vi "mightex.vi"() -> ()   [LabVIEW 2016]
uses:
  lib/SSClassic_USBCamera_SDK.dll
panel:
  in  "sharp":i32 min=0 max=3
  in  "bright":i32=50 min=0 max=100
  in  "contrast":i32=50 min=0 max=100
  in  "gamma":i32=10 min=1 max=20
  in  "Gain?":bool
  in  "Blue Gain":i32(slide)=17 scale=1.0..64.0
  in  "Green Gain":i32(slide)=16 scale=1.0..64.0
  in  "Red Gain":i32(slide)=20 scale=1.0..64.0
  out "new picture":picture
  out "Spectrum":u8[](graph)
  out "?":u8[](array[numeric])
  in  "STOP":bool
  in  "Exposure Time:":dbl(slide) scale=1.0..100.0
  out "ET Labelµ":dbl format="%#_3g"
  out "OK to run":bool
  out "SerialNo:":string
  out "ModuleNo:":string
  # "(ms )"
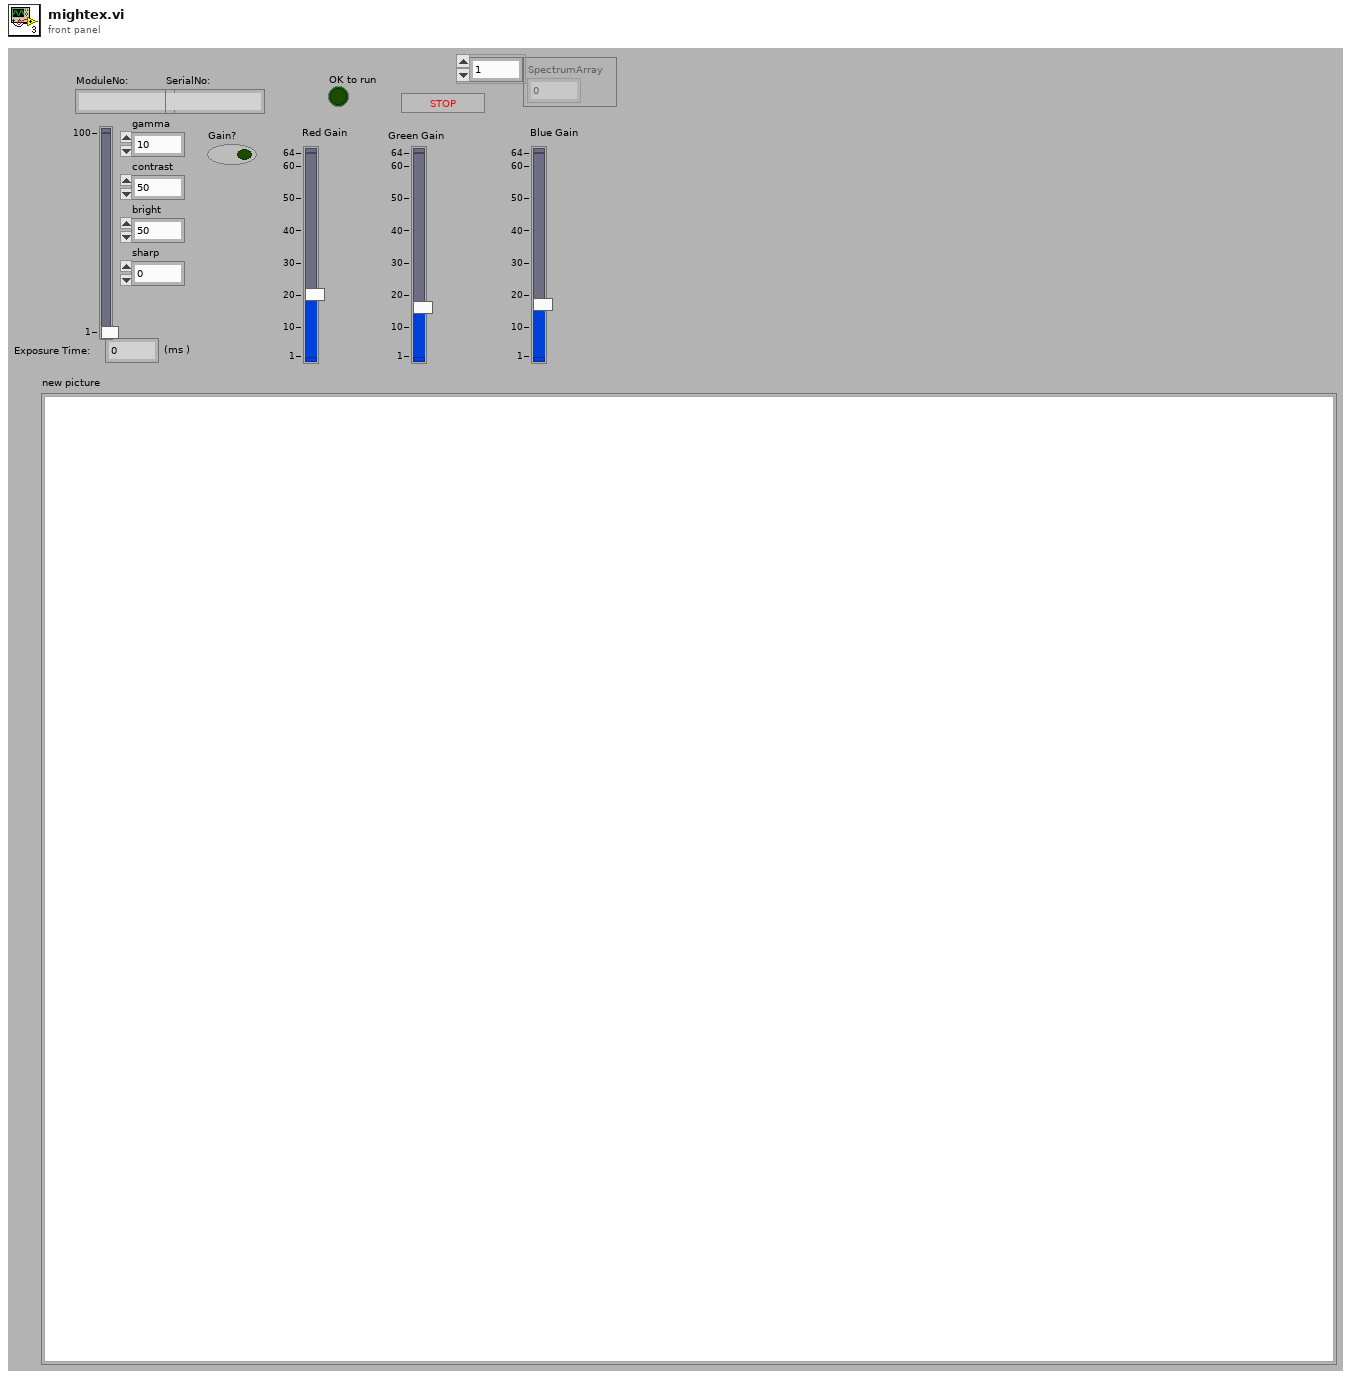
[diagram p1: front panel]
types:
  T1 = typedef "imagedata.ctl" = cluster{"image type":i32, "image depth":i32, "image":u8[], "mask":u8[], "colors":u32[], "Rectangle":cluster{"left":i16, "top":i16, "right":i16, "bottom":i16}}
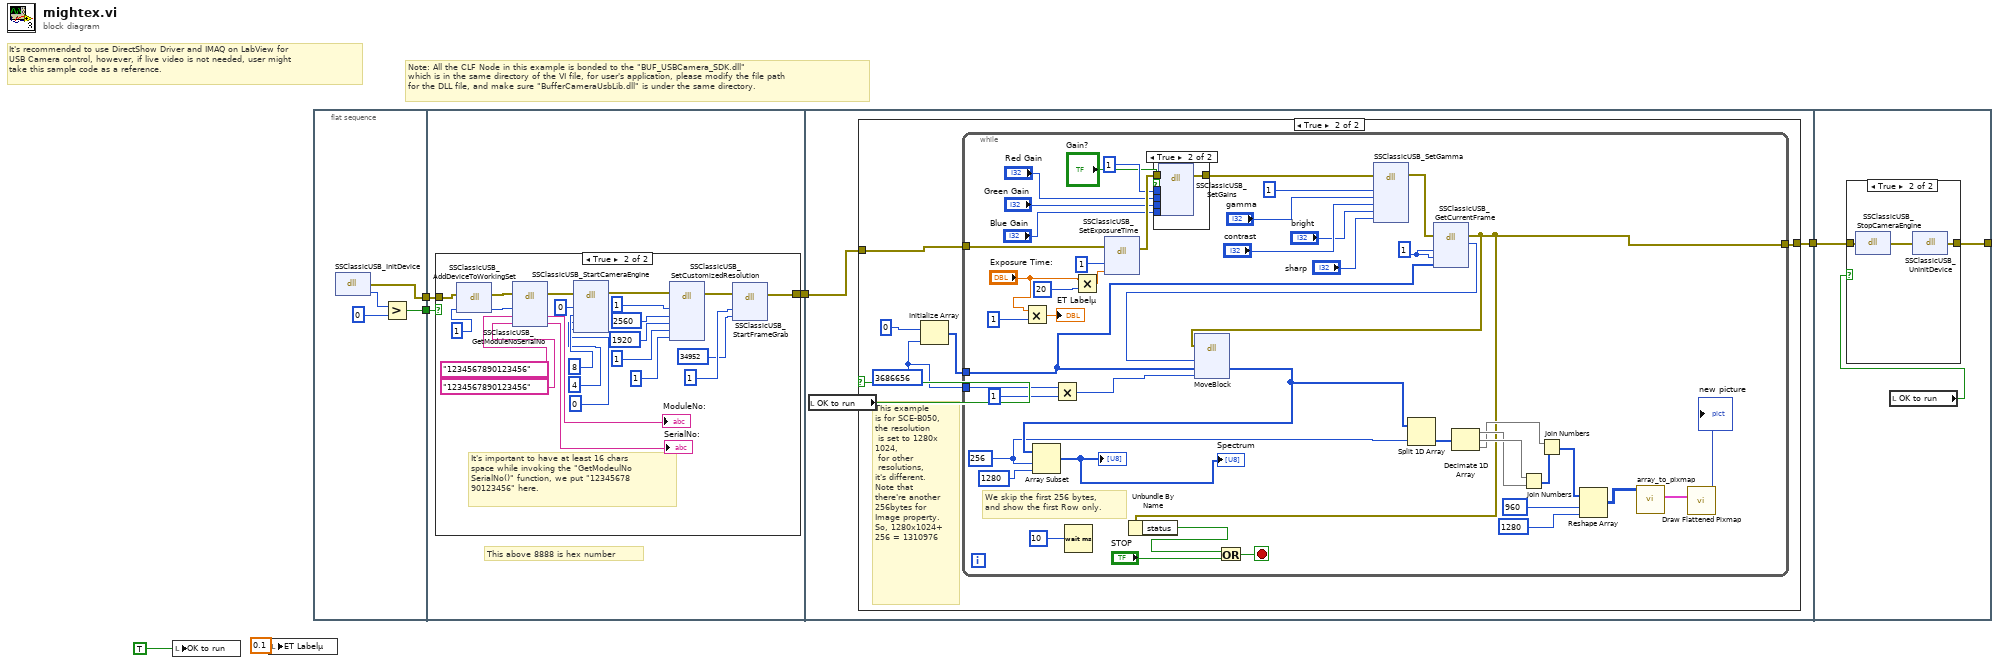
[diagram p0: block diagram]
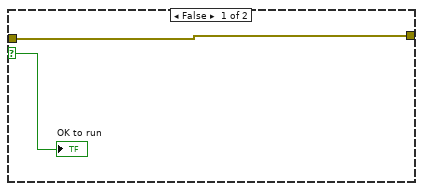
[diagram p2: hidden frame]
diagram:
  # "It's recommended to use DirectShow Driver and IMAQ on LabView for\nUSB Camera control, however, if live video is not needed, user might\ntake this sample code as a reference."
  # "Note: All the CLF Node in this example is bonded to the \"BUF_USBCamera_SDK.dll\" \nwhich is in the same directory of the VI file, for user's application, please modify the file path\nfor the DLL file, and make sure \"BufferCameraUsbLib.dll\" is under the same directory."
  n1 = local write "OK to run"(TRUE) -> ()
  n2 = local write "ET Labelµ"(0.1) -> ()
  n3 = flat-sequence {
    tunnel: [w8] -> w6
    tunnel: [w7] -> w5
    tunnel: w6 -> [w13]
    tunnel: w5 -> [w12]
    tunnel: [w11] -> w3
    tunnel: w3 -> [w40]
    tunnel: [w39] -> w2
    tunnel: w2 -> [w103]
    tunnel: [w102] -> _
    frame #0 {
      n4 = dll-call lib="D:/All users/PoSheng/src/lib/SSClassic_USBCamera_SDK.dll" fn="SSClassicUSB_InitDevice" ("CCD_USBCamera_SDK.dll:CCDUSB_InitDevice")() -> (error out=w7:errorcluster, "ReturnValue"=w10:u32)  [unwired: 3 in, 1 out]
      n5 = Greater?(x=w10, y=0) -> (0:w8:bool)
    }
    frame #1 {
      # "This above 8888 is hex number"
      n6 = case shown="True" w13 {
        selector: w13 -> [w15 _]
        tunnel: w12 -> [w14 w38]
        tunnel: [w14 w31] -> w11
        frame False {
          "OK to run" <- w15
        }
        frame True {
          # "It's important to have at least 16 chars\nspace while invoking the \"GetModeulNo\nSerialNo()\" function, we put \"12345678\n90123456\" here."
          n7 = dll-call lib="D:/All users/PoSheng/src/lib/SSClassic_USBCamera_SDK.dll" fn="SSClassicUSB_AddDeviceToWorkingSet" ("CCD_USBCamera_SDK.dll:CCDUSB_AddDeviceToWorkingSet")(error in=w38, "Arg1"=1) -> (error out=w37:errorcluster, "Arg1"=w35:i32)  [unwired: 3 in, 1 out]
          n8 = dll-call lib="D:/All users/PoSheng/src/lib/SSClassic_USBCamera_SDK.dll" fn="SSClassicUSB_GetModuleNoSerialNo" ("CCD_USBCamera_SDK.dll:CCDUSB_GetModuleNoSerialNo")(error in=w37, "Arg1"=w35, "Arg2"="1234567890123456", "Arg3"="1234567890123456") -> (error out=w33:errorcluster, "Arg2"=→"ModuleNo:":string, "Arg3"=→"SerialNo:":string)  [unwired: 4 in, 1 out]
          n9 = dll-call lib="D:/All users/PoSheng/src/lib/SSClassic_USBCamera_SDK.dll" fn="SSClassicUSB_StartCameraEngine" ("CCD_USBCamera_SDK.dll:CCDUSB_StartCameraEngine")(error in=w33, "Arg1"=0, "Arg2"=8, "Arg3"=4, "Arg4"=0) -> (error out=w26:errorcluster)  [unwired: 7 in, 1 out]
          n10 = dll-call lib="D:/All users/PoSheng/src/lib/SSClassic_USBCamera_SDK.dll" fn="SSClassicUSB_SetCustomizedResolution" ("BUF_USBCamera_SDK.dll:BUFUSB_SetCustomizedResolution")(error in=w26, "Arg1"=1, "Arg2"=2560, "Arg3"=1920, "Arg4"=1, "Arg5"=u32 1) -> (error out=w25:errorcluster)  [unwired: 8 in, 1 out]
          n11 = dll-call lib="D:/All users/PoSheng/src/lib/SSClassic_USBCamera_SDK.dll" fn="SSClassicUSB_StartFrameGrab" ("CCD_USBCamera_SDK.dll:CCDUSB_StartFrameGrab")(error in=w25, "Arg1"=1, "Arg2"=34952) -> (error out=w31:errorcluster)  [unwired: 5 in, 1 out]
        }
      }
    }
    frame #2 {
      n12 = local read "OK to run"() -> (w41:bool)
      n13 = case shown="True" w41 {
        tunnel: w40 -> [w42 w47]
        tunnel: [w42 w46] -> w39
        frame False {
        }
        frame True {
          w44 = 3686656 ("dimension size")
          # "This example\nis for SCE-B050,\nthe resolution\n is set to 1280x\n1024,\n for other  \n resolutions,\nit's different.\nNote that\nthere're another\n256bytes for\nImage property.\nSo, 1280x1024+\n256 = 1310976"
          n14 = Initialize Array ("初始化数组")(u8 0, w44) -> (w45:u8[])
          n15 = while {
            tunnel: w47 -> [w82]
            tunnel: [w62] -> w46
            tunnel: w45 -> [w76]
            tunnel: w44 -> [w80]
            stop <- w92 stop-if-true
            w55 = 256 ("y")
            w75 = 1
            # "We skip the first 256 bytes,\nand show the first Row only."
            n16 = Multiply(x="Exposure Time:", y=1) -> (x*y=→"ET Labelµ":dbl)
            n17 = Multiply(x=w80, y=1) -> (x*y=w79:i32)
            n18 = Wait (ms)(milliseconds to wait=10) -> ()  [unwired: 1 out]
            n19 = Multiply(x="Exposure Time:", y=20) -> (x*y=w85:dbl)
            n20 = dll-call lib="D:/All users/PoSheng/src/lib/SSClassic_USBCamera_SDK.dll" fn="SSClassicUSB_SetExposureTime" ("CCD_USBCamera_SDK.dll:CCDUSB_SetExposureTime")(error in=w82, "Arg1"=1, "Arg2"=w85) -> (error out=w61:errorcluster)  [unwired: 5 in, 1 out]
            n21 = case shown="True" "Gain?" {
              tunnel: w61 -> [w94 w100]
              tunnel: [w94 w99] -> w54
              tunnel: 1 ("deviceID") -> [_ w98]
              tunnel: "Red Gain" -> [_ w97]
              tunnel: "Green Gain" -> [_ w96]
              tunnel: "Blue Gain" -> [_ w95]
              frame False {
              }
              frame True {
                n22 = dll-call lib="D:/All users/PoSheng/src/lib/SSClassic_USBCamera_SDK.dll" fn="SSClassicUSB_SetGains" ("CCD_USBCamera_SDK.dll:CCDUSB_SetExposureTime")(error in=w100, "deviceID"=w98, "redGain"=w97, "greenGain"=w96, "blueGain"=w95) -> (error out=w99:errorcluster)  [unwired: 7 in, 1 out]
              }
            }
            n23 = dll-call lib="D:/All users/PoSheng/src/lib/SSClassic_USBCamera_SDK.dll" fn="SSClassicUSB_SetGamma" ("CCD_USBCamera_SDK.dll:CCDUSB_GetCurrentFrame")(error in=w54, "deviceID"=1, "gamma"="gamma", "contrast"="contrast", "bright"="bright", "sharp"="sharp") -> (error out=w53:errorcluster)  [unwired: 8 in, 1 out]
            n24 = dll-call lib="D:/All users/PoSheng/src/lib/SSClassic_USBCamera_SDK.dll" fn="SSClassicUSB_GetCurrentFrame" ("CCD_USBCamera_SDK.dll:CCDUSB_GetCurrentFrame")(error in=w53, "Arg1"=w75, "Arg2"=w75, "Arg3"=w76) -> (error out=w62:errorcluster, "ReturnValue"=w89:i64)  [unwired: 5 in, 1 out]
            n25 = Unbundle By Name(w62) -> ("status"=w91:bool)
            n26 = dll-call lib="LabVIEW" fn="MoveBlock"(error in=w62, "src"=w89, "dst"=w76, "size"=w79) -> ("dst"=w67:u8[])  [unwired: 5 in, 2 out]
            n27 = Array Subset(array=w67, index=w55, length=1280 ("y")) -> (→"?" →"Spectrum":u8[])
            n28 = Or(x=w91, y="STOP") -> (x .or. y?=w92:bool)
            n29 = Split 1D Array(array=w67, index=w55) -> (second subarray=w74:u8[])  [unwired: 1 out]
            n30 = Decimate 1D Array(w74) -> (w71:u8[], w72:u8[], w63:u8[])
            n31 = Join Numbers(hi=w72, lo=w71) -> ((hi.lo)=w73:u16[])
            n32 = Join Numbers(hi=w63, lo=w73) -> ((hi.lo)=w70:u32[])
            n33 = Reshape Array(w70, 960 ("dimension size"), 1280 ("dimension size")) -> (w66:u32[][])
            n34 = call "array_to_pixmap.vi"("photoarray"=w66) -> ("pixmap out"=w65:T1)  [unwired: 9 in, 1 out]
            n35 = call <vilib>:"Draw Flattened Pixmap.vi"("image data"=w65) -> ("new picture"=→"new picture":picture)  [unwired: 8 in]
          }
        }
      }
    }
    frame #3 {
      n36 = local read "OK to run"() -> (w101:bool)
      n37 = case shown="True" w101 {
        tunnel: w103 -> [w104 w107]
        tunnel: [w104 w105] -> w102
        frame False {
        }
        frame True {
          n38 = dll-call lib="D:/All users/PoSheng/src/lib/SSClassic_USBCamera_SDK.dll" fn="SSClassicUSB_StopCameraEngine" ("CCD_USBCamera_SDK.dll:CCDUSB_StopCameraEngine")(error in=w107) -> (error out=w106:errorcluster)  [unwired: 3 in, 1 out]
          n39 = dll-call lib="D:/All users/PoSheng/src/lib/SSClassic_USBCamera_SDK.dll" fn="SSClassicUSB_UnInitDevice" ("CCD_USBCamera_SDK.dll:CCDUSB_UnInitDevice")(error in=w106) -> (error out=w105:errorcluster)  [unwired: 3 in, 1 out]
        }
      }
    }
  }
